vi "555组成施密特电路.vi"() -> ()   [LabVIEW 2018]
panel:
  out "XY图":cluster{dbl[], i16[]}(graph)
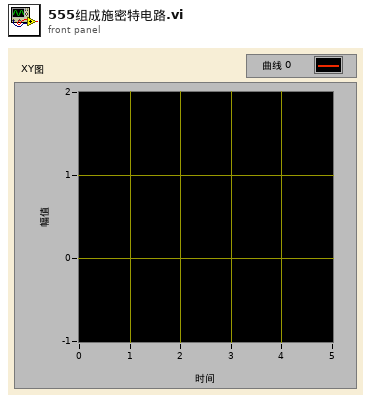
[diagram p1: front panel]
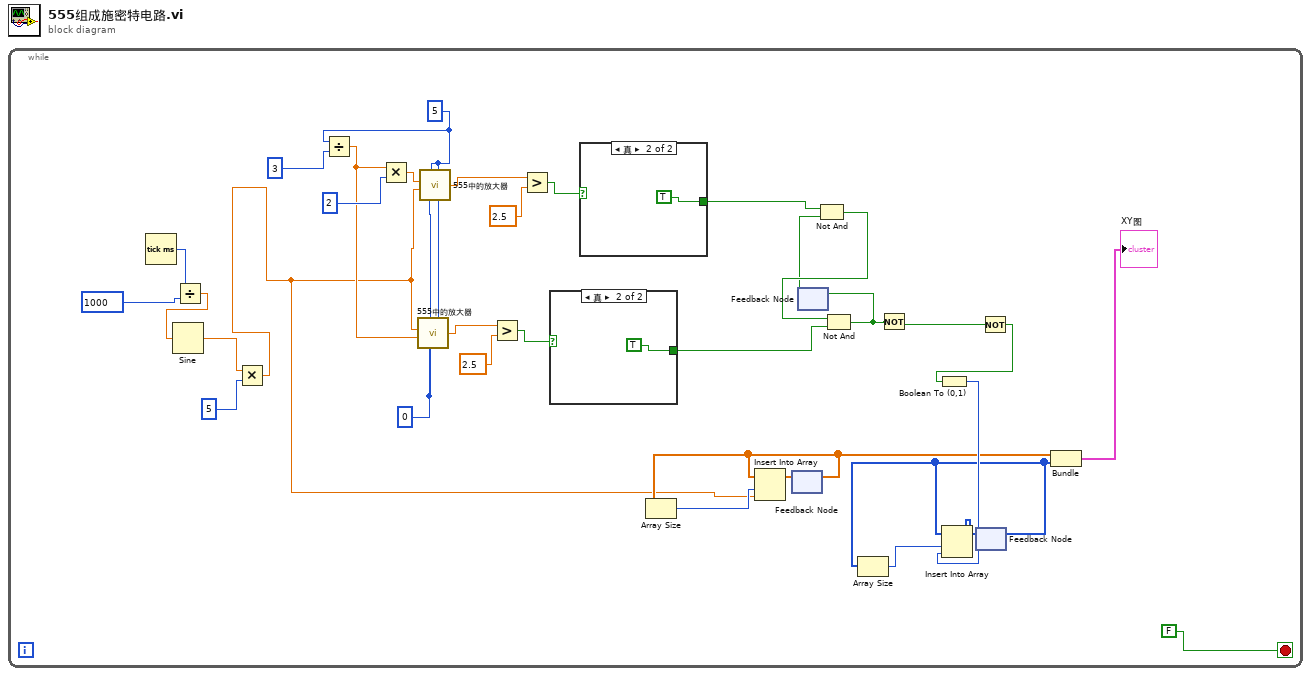
[diagram p0: block diagram]
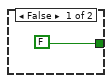
[diagram p2: hidden frame]
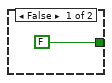
[diagram p3: hidden frame]
diagram:
  n1 = while {
    stop <- FALSE stop-if-true
    w34 = 0
    w20 = 5
    n2 = Tick Count (ms)() -> (millisecond timer value=w3:u32)
    n3 = Divide(x=w3, y=1000) -> (x/y=w1:dbl)
    n4 = Sine(x=w1) -> (sin(x)=w4:dbl)
    n5 = Multiply(x=w4, y=5) -> (x*y=w5:dbl)
    n6 = Divide(x=w20, y=3) -> (x/y=w18:dbl)
    n7 = Multiply(x=w18, y=2) -> (x*y=w17:dbl)
    n8 = call "555中的放大器.vi"("VCC"=w20, "IN+"=w5, "IN--"=w18, "--VCC"=w34) -> ("OUT"=w28:dbl)  [unwired: 4 in]
    n9 = call "555中的放大器.vi"("VCC"=w20, "IN+"=w17, "IN--"=w5, "--VCC"=w34) -> ("OUT"=w33:dbl)  [unwired: 4 in]
    n10 = Greater?(x=w28, y=2.5) -> (0:w29:bool)
    n11 = Greater?(x=w33, y=2.5) -> (0:w31:bool)
    n12 = case shown="真" w29 {
      tunnel: [FALSE TRUE] -> w26
      frame False {
      }
      frame True {
      }
    }
    n13 = case shown="真" w31 {
      tunnel: [FALSE TRUE] -> w27
      frame False {
      }
      frame True {
      }
    }
    n14 = feedback #1() -> (w9:dbl[])  [unwired: 1 in]
    n15 = Array Size(array=w9) -> (size(s)=w16:i32)
    n16 = Insert Into Array(array=w9, index=w16, new element=w5) -> (w10:dbl[])
    n17 = feedback-in #1(w10) -> ()
    n18 = feedback #2() -> (w24:bool)  [unwired: 1 in]
    n19 = Not And(1:w24, 2:w27) -> (0:w25:bool)
    n20 = Not And(1:w26, 2:w25) -> (0:w23:bool)
    n21 = feedback-in #2(w23) -> ()
    n22 = Not(x=w23) -> (.not. x?=w22:bool)
    n23 = feedback #3() -> (w7:i16[])  [unwired: 1 in]
    n24 = Array Size(array=w7) -> (size(s)=w13:i32)
    n25 = Not(x=w22) -> (.not. x?=w15:bool)
    n26 = Boolean To (0,1)(Boolean=w15) -> (0, 1=w14:i16)
    n27 = Insert Into Array(array=w7, index=w13, new element=w14) -> (w8:i16[])
    n28 = feedback-in #3(w8) -> ()
    n29 = Bundle(w9, w7) -> (→"XY图":cluster{dbl[], i16[]})  [unwired: 1 in]
  }
